vi "getSpec.vi"(10 "specData":string[][](array[string]), 11 "itemName":string) -> (2 "lowerLimit":dbl[](array[numeric]), 3 "upperLimit":dbl[](array[numeric]))   [LabVIEW 2011]
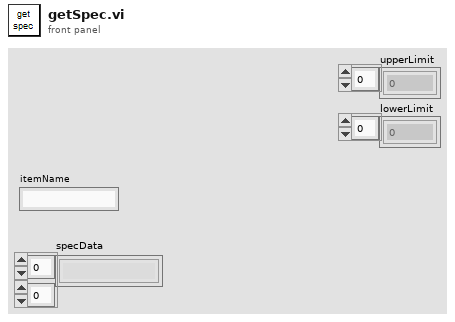
[diagram p1: front panel]
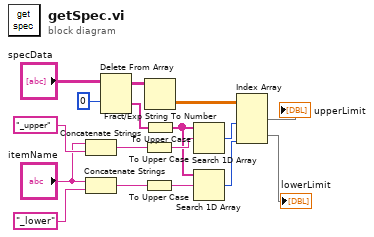
[diagram p0: block diagram]
diagram:
  n1 = Concatenate Strings("itemName", "_upper" ("字符串")) -> (w11:string)
  n2 = Concatenate Strings("itemName", "_lower" ("字符串")) -> (w10:string)
  n3 = Delete From Array(array="specData", index (row)=0 ("索引 (行)")) -> (deleted portion=w15:string[], array with subset deleted=w4:string[][])  [unwired: 2 in]
  n4 = To Upper Case(1:w11) -> (0:w9:string)
  n5 = To Upper Case(1:w10) -> (0:w8:string)
  n6 = Fract/Exp String To Number(string=w4) -> (number=w3:dbl[][])  [unwired: 3 in, 1 out]
  n7 = To Upper Case(1:w15) -> (0:w7:string[])
  n8 = Search 1D Array(1D array=w7, element=w9) -> (index of element=w6:i32)  [unwired: 1 in]
  n9 = Search 1D Array(1D array=w7, element=w8) -> (index of element=w5:i32)  [unwired: 1 in]
  n10 = Index Array(array=w3, index (col) #1=w6, index (col) #2=w5) -> (element #1=→"upperLimit":dbl[], element #2=→"lowerLimit":dbl[])  [unwired: 2 in]
